vi "SMC_Errors.vi"(9 "Error Code":i32=2000, 11 "Language":enum16{"Deutsch", "English"}(ring)) -> (1 "Answer":string="nicht definierter Befehl")   [LabVIEW 2012, in "Micos_uic.lvlib"]
uses:
  Micos_uic.lvlib
panel:
  in  "Meldungen":string[][](array[string])=[["1", "interner Fehler", "internal Error"], ["2", "interner Fehler", "internal Error"], ["3", "interner Fehler", "internal Error"], ["4", "interner Fehler", "internal Error"], ["5", "MR-Fehler", "MR Error"], ["6", "MR-Fehler", "MR Error"], ["7", "MR-Fehler", "MR Error"], ["8", "Übertragungsfehler", "transfer error"], ["9", "interner Fehler", "internal Error"], ["1001", "Falscher Parametertyp", "wrong parameter type"], ["1002", "zu wenige Parameter", "not enough parameters for the command on the stack"], ["1003", "Wertebereich des Parameters überschritten", "value range of the parameter is crossed"], ["1004", "Verfahrbereich sollte überschritten werden", "process range should be crossed"], ["1005", "Fahrfehler aufgetreten (closed loop)", "reserved"], ["1006", "falscher parameterwert bei restore", "wrong parameter value at the restore operation detected"], ["1007", "ungültiger Parameterwert", "invalid parameter value"], ["1008", "zu wenige Parameter auf dem Stack", "not enough parameters on the stack"], ["1009", "zu wenig Platz auf dem Stack für Parameter", "not enough room on the stack for all parameters"], ["1010", "kein Speicher mehr frei", "no more available memory"], ["1011", "keine Kette selektiert", "no chain selected"], ["1012", "keine Position in der Kette angefahren", "no next position in the selected chain"], ["1013", "keine Position in der Kette vorhanden", "no position in the current chain available"], ["1014", "Position in der Kette nicht vorhanden", "index in the chain not available"], ["1015", "Parameterwerte außerhalb des Tischverfahrweges", "parameter values out of the possible limits"], ["1016", "In der Kette wurde der kleinste Index überschritten", "in the chain the least index is crossed"], ["1017", "In der Kette wurde der größte Index überschritten", "in the chain the greatest index is crossed"], ["1018", "Kantenzähler ist 0", "reserved"], ["1100", "Division durch 0", "division by zero"], ["2000", "nicht definierter Befehl", "undefined command"], ["2011", "Schrittfehler X-Achse aufgetreten", "step error in x-axis appeared"], ["2012", "Schrittfehler Y-Achse aufgetreten", "step error in y-axis appeared"], ["2013", "Schrittfehler X- und Y-Achse aufgetreten", "step error in x and y-axis appeared"], ["2014", "Schrittfehler Z-Achse aufgetreten", "step error in z-axis appeared"], ["2015", "Schrittfehler X- und Z-Achse aufgetreten", "step error in x and z-axis appeared"], ["2016", "Schrittfehler Y- und Z-Achse aufgetreten", "step error in y and z-axis appeared"], ["2017", "Schrittfehler X-, Y- und Z-Achse aufgetreten", "step error in x, y and z-axis appeared"], ["4000", "Selbsttestfehler aufgetreten", "self test error appeared"], ["7001", "I/O Port nicht vorhanden", "I/O port not present"], ["7002", "mode = 1 nur für die serielle Schnittstelle erlaubt", "mode = 1 only for the serial line allowed"], ["9000", "Fehler beim Empfang über die serielle Schnittstelle", "reserved"], ["9001", "Interner Fehler beim Empfang über die serielle Schnittstelle", "reserved"]]
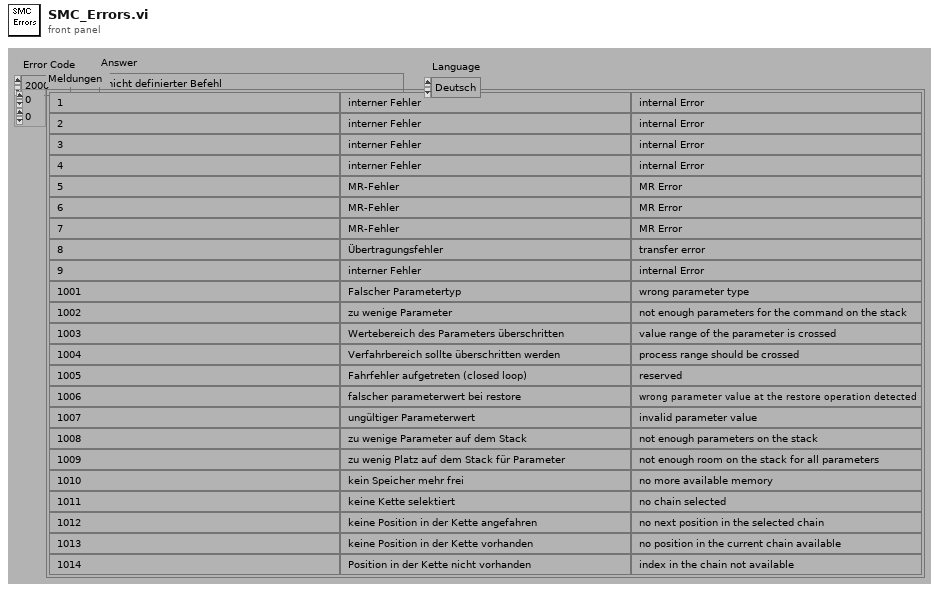
[diagram p1: front panel]
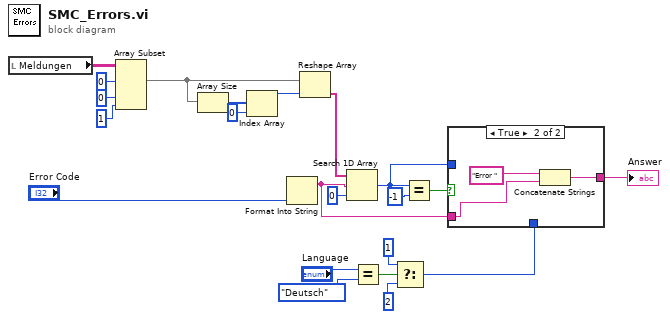
[diagram p0: block diagram]
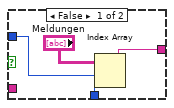
[diagram p2: hidden frame]
diagram:
  n1 = local read "Meldungen"() -> (w16:string[][])
  n2 = Array Subset "Array Subset"(array=w16, index (row)=0, index (col)=0, length (col)=1) -> (w12:string[][])  [unwired: 1 in]
  n3 = Array Size(array=w12) -> (size(s)=w11:i32[])
  n4 = Index Array(array=w11, index=0) -> (element=w9:i32)
  n5 = Format Into String("Error Code") -> (resulting string=w7:string)  [unwired: 3 in, 1 out]
  n6 = Reshape Array "Reshape Array"(w12, w9) -> (w8:string[])
  n7 = Search 1D Array(1D array=w8, element=w7, start index (0)=0) -> (index of element=w18:i32)
  n8 = Equal?(x="Language", y=enum16{"Deutsch", "English"}."Deutsch") -> (x = y?=w4:bool)
  n9 = Select(t=1, s=w4, f=2) -> (s? t:f=w3:i32)
  n10 = Equal?(x=w18, y=-1) -> (x = y?=w20:bool)
  n11 = case shown="True" w20 {
    tunnel: [w24 w29] -> w19
    tunnel: w18 -> [w26 _]
    tunnel: w7 -> [_ w27]
    tunnel: w3 -> [w23 _]
    frame False {
      n12 = Index Array(array="Meldungen", index (row)=w26, index (col)=w23) -> (element=w24:string)
    }
    frame True {
      n13 = Concatenate Strings("Error ", w27) -> (w29:string)
    }
  }
  "Answer" <- w19
